vi "uintUintToString.vi"(8 "Error in (no error)":errorcluster, 11 "Uint in":refnum<class "UintClass.lvclass">) -> (0 "Error out":errorcluster, 2 "String":string, 3 "Uint out":refnum<class "UintClass.lvclass">)   [LabVIEW 2011, in "UintClass.lvclass"]
uses:
  UintClass.lvclass
  UintClass.lvclass/UintClass.ctl
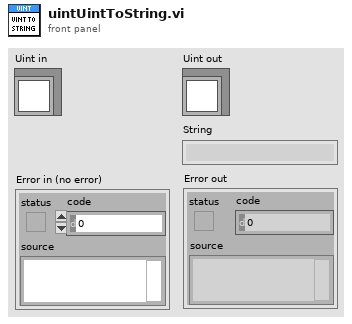
[diagram p1: front panel]
types:
  T1 = typedef "UintClass.lvclass/enumBase.ctl" = u16
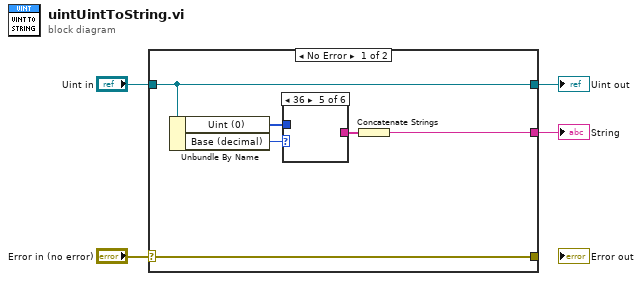
[diagram p0: block diagram]
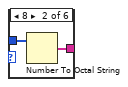
[diagram p3: hidden frame]
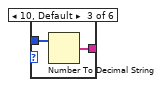
[diagram p4: hidden frame]
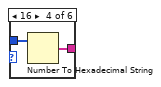
[diagram p5: hidden frame]
diagram:
  n1 = case shown="No Error" "Error in (no error)" {
    selector: "Error in (no error)" -> [w10 w17]
    tunnel: [w10 w17] -> _
    tunnel: [w9 w18] -> w3
    tunnel: "Uint in" -> [w9 w18]
    tunnel: [w6 _] -> w2
    frame No Error {
      n2 = Unbundle By Name(w9) -> ("Uint (0)"=w8:u8[], "Base (decimal)"=w5:T1)
      n3 = case shown="36" w5 {
        tunnel: w8 -> [_ w12 w14 w16 _ _]
        tunnel: [_ w11 w13 w15 _ _] -> w7
        frame 2 {
        }
        frame 8 {
          n4 = Number To Octal String(2:w12) -> (0:w11:string[])  [unwired: 1 in]
        }
        frame 10, Default {
          n5 = Number To Decimal String(number=w14) -> (decimal integer string=w13:string[])  [unwired: 1 in]
        }
        frame 16 {
          n6 = Number To Hexadecimal String(2:w16) -> (0:w15:string[])  [unwired: 1 in]
        }
        frame 36 {
        }
        frame 64 {
        }
      }
      n7 = Concatenate Strings(w7) -> (w6:string)
    }
    frame Error {
    }
  }
  "Uint out" <- w3
  "String" <- w2
